vi "字符检测模板匹配.vi"(0 "Image In":T6, 1 "Image Dst":T6, 2 "ROI Descriptor (Geometric Matching 1)":T5={"Global Rectangle"=[20, 20, 890, 1177], "Contours"=[{"ID"=enum."External", "Type"=3, "Coordinates"=[20, 20, 890, 1177]}]} {"Contours"."Type" items=["No Selection", "Point", "Line", "Rectangle", "Oval", "Polygon", "Freehand Region", "Annulus", "Unused2", "Unused3", "Broken Line", "Freehand Line", "Rotated Rectangle"]}, 3 "Settings (Geometric Matching 1)":T4={"Curve Parameters"={"Extraction Mode"=0, "Edge Threshold"=75, "Edge Filter Size"=1, "Min Length"=25, "Row Search Step Size"=15, "Col Search Step Size"=15, "Max Endpoint Gap"=10, "Closed"=FALSE, "Subpixel"=FALSE}, "Match Mode"={"Rotation"=TRUE, "Scale"=FALSE, "Occlusion"=TRUE, "Reserved 1"=FALSE, "Reserved 2"=FALSE, "Reserved 3"=FALSE}, "Range Settings"=[{"Match Constraints"=0, "Min"=0.0, "Max"=360.0}, {"Match Constraints"=2, "Min"=0.0, "Max"=25.0}], "Number of Matches"=1, "Minimum Match Score"=800.0, "SubPixel Accuracy"=FALSE, "Adv. Geometric Match Options 2"=[{"Setup Data Item"=21, "Item Value"=0.0}, {"Setup Data Item"=22, "Item Value"=1.0}]} {"Curve Parameters"."Extraction Mode" items=["Normal", "Uniform Regions"]; "Curve Parameters"."Edge Filter Size" items=["Fine", "Normal", "Contour Tracing"]; "Curve Parameters"."Max Endpoint Gap" min=0; "Curve Parameters"."Col Search Step Size" min=1 max=255 step=1; "Curve Parameters"."Row Search Step Size" min=1 max=255 step=1; "Curve Parameters"."Min Length" min=0; "Curve Parameters"."Edge Threshold" min=1 max=350 step=1; "Range Settings"."Max" format="%.2f"; "Range Settings"."Min" format="%.2f"; "Range Settings"."Match Constraints" items=["Rotation Angle (degrees)", "Scale Factor (%)", "Occlusion (%)"]; "Adv. Geometric Match Options 2"."Setup Data Item" items=["Curve Extraction Mode", "Curve Edge Threshold", "Curve Edge Filter Size", "Min Curve Length", "Curve Row Search Step Size", "Curve Col Search Step Size", "Curve Max Endpoint Gap", "Extract Closed Curves", "Enable Subpixel Curve Extraction", "Enable Correlation Score", "Enable Subpixel Accuracy", "Subpixel Iterations", "Subpixel Tolerance", "Initial Match List Length", "Enable Target Template Curve Score", "Min Match Separation Distance", "Min Match Separation Angle", "Min Match Separation Scale", "Max Match Overlap", "Enable Coarse Result", "Enable Calibration Support", "Enable Contrast Reversal", "Search Strategy", "Refinement Match Factor", "Subpixel Match Factor"]}, 4 "Template File Path (Geometric Matching 1)":path=path "D:/Inspect System/Source Code/SubVIs/字符检测VI/aaaa.png", 5 "Reference System":T1 {"Axis Reference" items=["Direct", "Indirect"]; "Angle (deg)" format="%.2f"; "Origin"."Y" format="%.2f"; "Origin"."X" format="%.2f"}, 7 "error in":errorcluster) -> (20 "Image Out":T6, 21 "Matches (Geometric Matching 1)":T8[](array[typedef]) {"Correlation Score" format="%.2f"; "Target Template Curve Score" format="%.2f"; "Template Target Curve Score" format="%.2f"; "Bounding Box"."y" format="%.2f"; "Bounding Box"."x" format="%.2f"; "Position"."y" format="%.2f"; "Position"."x" format="%.2f"; "Score" format="%.2f"; "Scale" format="%.2f"; "Angle" format="%.2f"; "Occlusion %" format="%.2f"}, 22 "Calibrated Matches (Geometric Matching 1)":T8[](array[typedef]) {"Correlation Score" format="%.2f"; "Target Template Curve Score" format="%.2f"; "Template Target Curve Score" format="%.2f"; "Bounding Box"."y" format="%.2f"; "Bounding Box"."x" format="%.2f"; "Position"."y" format="%.2f"; "Position"."x" format="%.2f"; "Score" format="%.2f"; "Scale" format="%.2f"; "Angle" format="%.2f"; "Occlusion %" format="%.2f"}, 23 "Number of Matches (Geometric Matching 1)":i32, 24 "Coordinate System Out (Set Coordinate System 1)":T7 {"Measurement System"."Axis Reference" items=["Direct", "Indirect"]; "Measurement System"."Angle (deg)" format="%.2f"; "Measurement System"."Origin"."Y" format="%.2f"; "Measurement System"."Origin"."X" format="%.2f"; "Reference System"."Axis Reference" items=["Direct", "Indirect"]; "Reference System"."Angle (deg)" format="%.2f"; "Reference System"."Origin"."Y" format="%.2f"; "Reference System"."Origin"."X" format="%.2f"}, 27 "error out":errorcluster)   [LabVIEW 2017]
doc: "Creates, edits, and runs vision algorithms using NI Vision Assistant.\n\nWhen you place this Express VI on the block diagram, NI Vision Assistant launches. Create an algorithm using the Vision Assistant processing functions. After you create an algorithm, you can select the controls and indicators that you want to be able to programmatically set in LabVIEW. Double-click the Vision Assistant Express VI to edit the algorithm."
uses:
  <vilib>/vision/Image Controls.llb/IMAQ Image.ctl
  <vilib>/vision/Pattern Matching.llb/IMAQ GM Match Report.ctl
  <vilib>/vision/Pattern Matching.llb/IMAQ Curve Parameters.ctl
  <vilib>/vision/Pattern Matching.llb/IMAQ Match Range Setting.ctl
panel:
  # "Range"
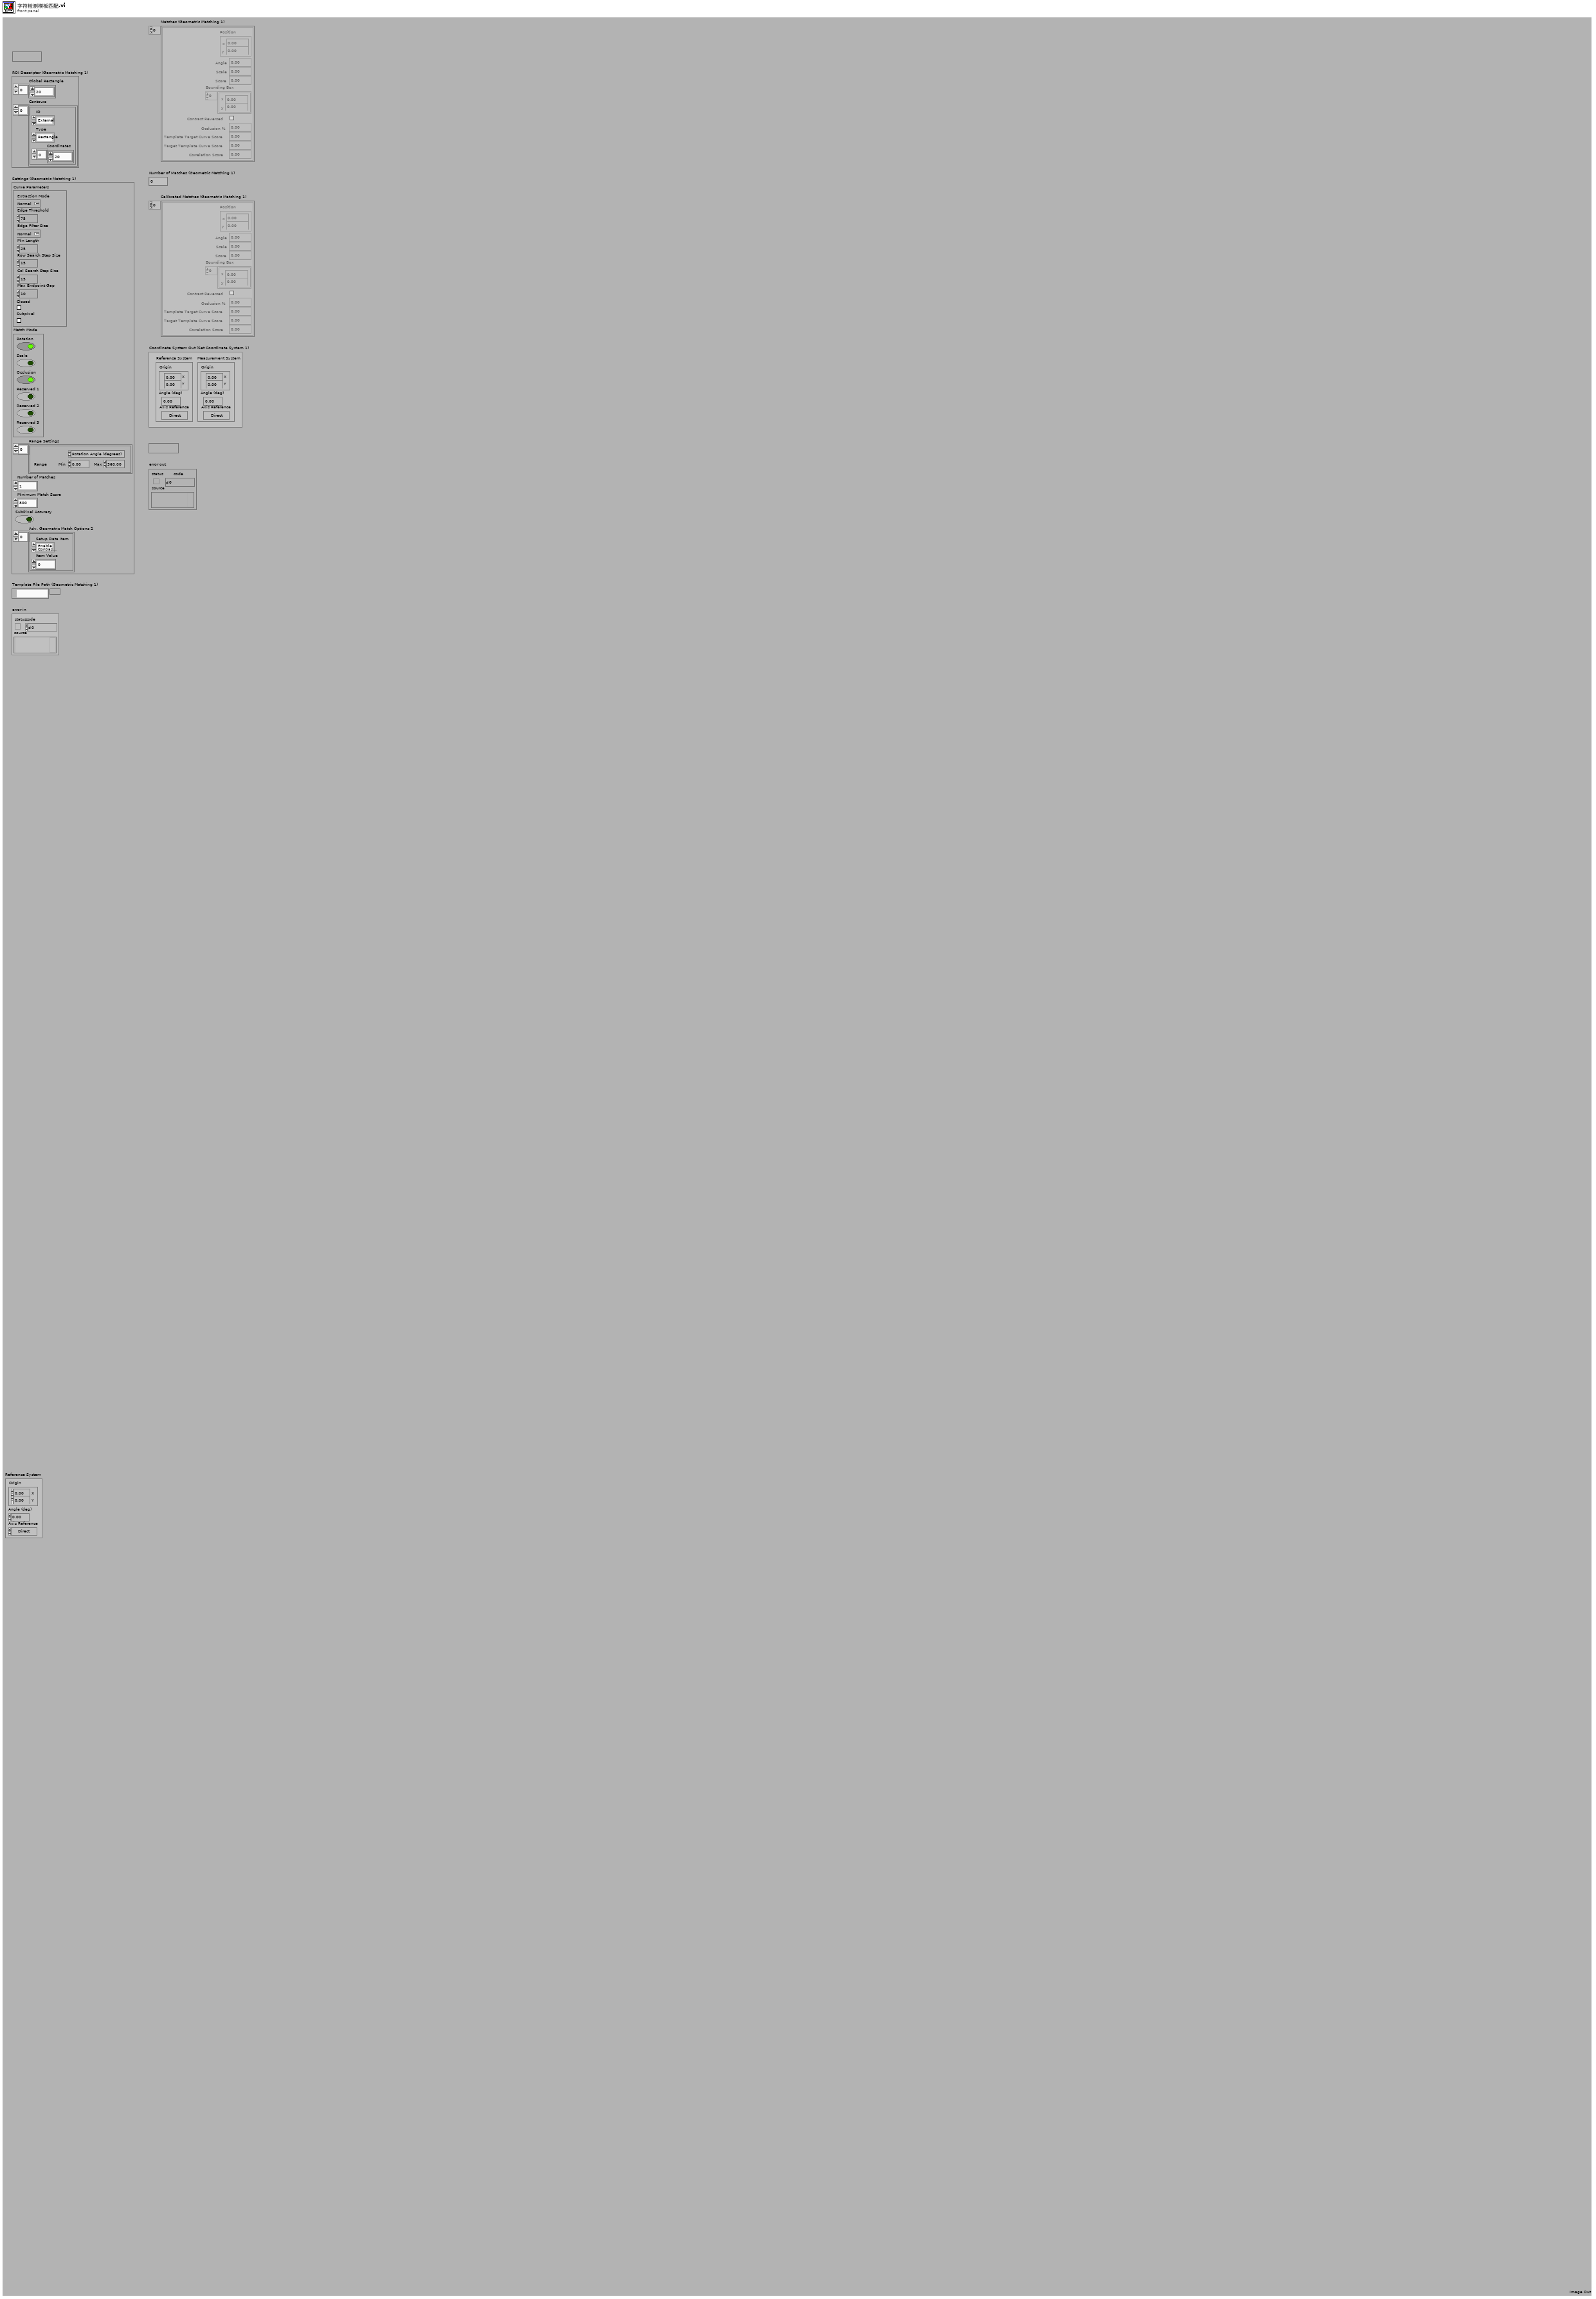
[diagram p1: front panel]
types:
  T1 = cluster{"Origin":cluster{"X":sgl, "Y":sgl}, "Angle (deg)":sgl, "Axis Reference":u32}
  T2 = typedef "IMAQ Curve Parameters.ctl" = cluster{"Extraction Mode":u32, "Edge Threshold":i32, "Edge Filter Size":u32, "Min Length":i32, "Row Search Step Size":i32, "Col Search Step Size":i32, "Max Endpoint Gap":i32, "Closed":bool, "Subpixel":bool}
  T3 = typedef "IMAQ Match Range Setting.ctl" = cluster{"Match Constraints":u32, "Min":dbl, "Max":dbl}
  T4 = cluster{"Curve Parameters":T2, "Match Mode":cluster{"Rotation":bool, "Scale":bool, "Occlusion":bool, "Reserved 1":bool, "Reserved 2":bool, "Reserved 3":bool}, "Range Settings":T3[], "Number of Matches":i32, "Minimum Match Score":sgl, "SubPixel Accuracy":bool, "Adv. Geometric Match Options 2":cluster{"Setup Data Item":u16, "Item Value":dbl}[]}
  T5 = cluster{"Global Rectangle":i32[], "Contours":cluster{"ID":enum32{"External", "Internal"}, "Type":u32, "Coordinates":i32[]}[]}
  T6 = typedef "IMAQ Image.ctl" = refnum<image>
  T7 = cluster{"Reference System":cluster{"Origin":cluster{"X":sgl, "Y":sgl}, "Angle (deg)":sgl, "Axis Reference":u32}, "Measurement System":cluster{"Origin":cluster{"X":sgl, "Y":sgl}, "Angle (deg)":sgl, "Axis Reference":u32}}
  T8 = typedef "IMAQ GM Match Report.ctl" = cluster{"Position":cluster{"x":sgl, "y":sgl}, "Angle":sgl, "Scale":sgl, "Score":sgl, "Bounding Box":cluster{"x":sgl, "y":sgl}[], "Contrast Reversed":bool, "Occlusion %":sgl, "Template Target Curve Score":sgl, "Target Template Curve Score":sgl, "Correlation Score":sgl}
  T9 = typedef "Image Type" = u32
  T10 = enum16{"Reset", "Update Coordinate System", "Get Coordinate System"}
  T11 = enum16{"Horizontal Motion", "Vertical Motion", "Horizontal and Vertical Motion", "Horizontal, Vertical and Angular Motion"}
  T12 = typedef "IMAQ Coordinate System" = cluster{"Reference System":cluster{"Origin":cluster{"X":sgl, "Y":sgl}, "Angle (deg)":sgl, "Axis Reference":u32}, "Measurement System":cluster{"Origin":cluster{"X":sgl, "Y":sgl}, "Angle (deg)":sgl, "Axis Reference":u32}}
  T13 = cluster{"Backup Image Name":string, "Coordinate System Out":T12}
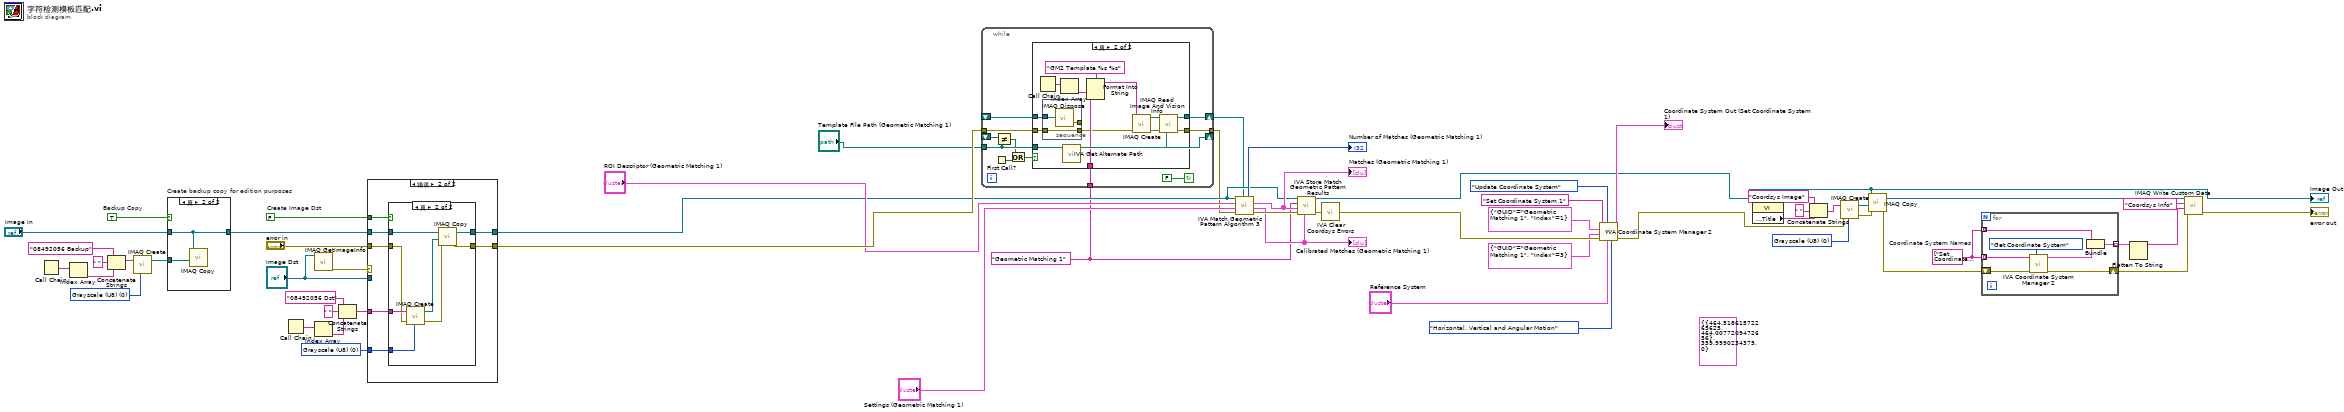
[diagram p0: block diagram]
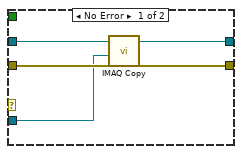
[diagram p3: hidden frame]
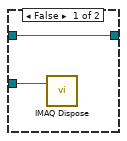
[diagram p5: hidden frame]
diagram:
  w5 = T9 0 items=["Grayscale (U8)", "Grayscale (I16)", "Grayscale (SGL)", "Complex (CSG)", "RGB (U32)", "HSL (U32)", "RGB (U64)", "Grayscale (U16)"] ("Image Type")
  w12 = string[] ["Set Coordinate System 1"]  # Coordinate System Names
  (unwired) T1 {"Origin"={"X"=464.51862, "Y"=464.00772}, "Angle (deg)"=359.99902, "Axis Reference"=0} ("Reference System")
  w29 = "Geometric Matching 1" ("Step Name")
  w38 = T9 0 items=["Grayscale (U8)", "Grayscale (I16)", "Grayscale (SGL)", "Complex (CSG)", "RGB (U32)", "HSL (U32)", "RGB (U64)", "Grayscale (U16)"] ("Image Dst Type")
  w39 = T9 0 items=["Grayscale (U8)", "Grayscale (I16)", "Grayscale (SGL)", "Complex (CSG)", "RGB (U32)", "HSL (U32)", "RGB (U64)", "Grayscale (U16)"] ("Image Type")
  w58 = TRUE  # Backup Copy
  w51 = FALSE  # Create Image Dst
  n1 = Call Chain() -> (call chain=w45:string[])
  n2 = Index Array(array=w45) -> (element=w44:string)  [unwired: 1 in]
  n3 = Concatenate Strings("08492056 Backup" ("Backup Image Name"), " ", w44) -> (w41:string)
  n4 = call "IMAQ Create"("Image Name"=w41, "Image Type"=w39) -> ("New Image"=w40:T6)  [unwired: 2 in, 2 out]
  n5 = case "Create backup copy for edition purposes" shown="真" w58 {
    tunnel: [w60 w62] -> w54
    tunnel: "Image In" -> [w60 w62]
    tunnel: w40 -> [w59 w61]
    frame False {
      n6 = call "IMAQ Dispose"("Image"=w59) -> ()  [unwired: 2 in, 4 out]
    }
    frame True {
      n7 = call "IMAQ Copy"("Image Dst"=w61, "Image Src"=w62) -> ()  [unwired: 1 in, 5 out]
    }
  }
  n8 = Call Chain() -> (call chain=w50:string[])
  n9 = call "IMAQ GetImageInfo"("Image"="Image Dst") -> ("error out"=w56:errorcluster)  [unwired: 1 in, 9 out]
  n10 = Index Array(array=w50) -> (element=w48:string)  [unwired: 1 in]
  n11 = Concatenate Strings("08492056 Dst" ("Image Dst Name"), " ", w48) -> (w46:string)
  n12 = case "条件结构" shown="错误" w56 {
    tunnel: [w67 w71] -> w31
    tunnel: [w66 w70] -> w52
    tunnel: w54 -> [w65 w72]
    tunnel: "error in" -> [w64 w68]
    tunnel: "Image Dst" -> [w63 _]
    tunnel: w46 -> [_ w74]
    tunnel: w38 -> [_ w73]
    tunnel: w51 -> [_ w69]
    frame No Error {
      n13 = call "IMAQ Copy"("error in (no error)"=w64, "Image Dst"=w63, "Image Src"=w65) -> ("error out"=w66:errorcluster, "Image Dst Out"=w67:T6)  [unwired: 3 out]
    }
    frame Error {
      n14 = case "条件结构" shown="真" w69 {
        tunnel: w74 -> [_ w84]
        tunnel: w73 -> [_ w83]
        tunnel: w72 -> [w76 w81]
        tunnel: [w76 w80] -> w71
        tunnel: [w75 w79] -> w70
        tunnel: w68 -> [w75 w77]
        frame False {
        }
        frame True {
          n15 = call "IMAQ Create"("Image Name"=w84, "Image Type"=w83, "error in (no error)"=w77) -> ("New Image"=w82:T6, "error out"=w78:errorcluster)  [unwired: 1 in, 1 out]
          n16 = call "IMAQ Copy"("error in (no error)"=w78, "Image Dst"=w82, "Image Src"=w81) -> ("error out"=w79:errorcluster, "Image Dst Out"=w80:T6)  [unwired: 3 out]
        }
      }
    }
  }
  n17 = while {
    shift-right: [w95] -> w27
    shift-left: _ -> [w94]
    tunnel: [w92] -> w28
    tunnel: w52 -> [w91]
    tunnel: "Template File Path (Geometric Matching 1)" -> [w88]
    tunnel: w29 -> [w90]
    shift-right: [w88] -> _
    shift-left: _ -> [w89]
    stop <- FALSE continue-if-true
    n18 = First Call?() -> (First Call?: T/F=w87:bool)
    n19 = Not Equal?(x=w89, y=w88) -> (x != y?=w86:bool)
    n20 = Or(x=w86, y=w87) -> (x .or. y?=w85:bool)
    n21 = case "条件结构" shown="真" w85 {
      tunnel: [w97 w109] -> w95
      tunnel: w94 -> [w97 w101]
      tunnel: [w96 w106] -> w92
      tunnel: w91 -> [w96 w102]
      tunnel: w90 -> [_ w103]
      tunnel: w88 -> [_ w100]
      frame False {
      }
      frame True {
        n22 = Call Chain() -> (call chain=w105:string[])
        n23 = stacked-sequence "层叠式顺序结构" {
          tunnel: w102 -> [w114]
          tunnel: w101 -> [w113]
          tunnel: [w114] -> w98
          tunnel: [w112] -> _
          frame #0 {
            n24 = call "IMAQ Dispose"("Image"=w113) -> ("error out"=w112:errorcluster)  [unwired: 2 in, 3 out]
          }
        }
        n25 = Index Array(array=w105) -> (element=w104:string)  [unwired: 1 in]
        n26 = call <vilib>:"IVA Get Alternate Path.vi"("Path In"=w100) -> ("Path Out"=w99:path)  [unwired: 10 out]
        n27 = Format Into String(format string="GM2 Template %s %s" ("Image Name"), w104, w103) -> (resulting string=w111:string)  [unwired: 2 in, 1 out]
        n28 = call "IMAQ Create"("Image Name"=w111, "error in (no error)"=w98) -> ("New Image"=w108:T6, "error out"=w107:errorcluster)  [unwired: 2 in, 1 out]
        n29 = call "IMAQ Read Image And Vision Info"("File Path"=w99, "error in (no error)"=w107, "Image"=w108) -> ("error out"=w106:errorcluster, "Image Out"=w109:T6)  [unwired: 1 in, 6 out]
      }
    }
  }
  n30 = call <vilib>:"IVA Match Geometric Pattern Algorithm 3.vi"("Template"=w27, "error in (no error)"=w28, "Settings"="Settings (Geometric Matching 1)", "ROI Descriptor"="ROI Descriptor (Geometric Matching 1)", "Image"=w31) -> ("error out"=w35:errorcluster, "Calibrated Matches"=w33:T8[], "Matches"=w34:T8[], "Number of Matches"=→"Number of Matches (Geometric Matching 1)":i32)  [unwired: 3 out]
  "Matches (Geometric Matching 1)" <- w34
  "Calibrated Matches (Geometric Matching 1)" <- w33
  n31 = call <vilib>:"IVA Store Match Geometric Pattern Results.vi"("Calibrated Matches"=w33, "error in (no error)"=w35, "Matches"=w34, "Step Name"=w29, "Image in"=w31) -> ("error out"=w26:errorcluster, "Image dup"=w2:T6)  [unwired: 5 out]
  "Image Out" <- w2
  n32 = call <vilib>:"IVA Clear Coordsys Errors.vi"("error in (no error)"=w26) -> ("error out"=w25:errorcluster)  [unwired: 10 in]
  n33 = call <vilib>:"IVA Coordinate System Manager 2.vi"("Mode"=T11."Horizontal, Vertical and Angular Motion", "Reference System"="Reference System", "Function"=T10."Update Coordinate System", "error in (no error)"=w25, "Angle ID"=cluster{"GUID":string, "Index":i32} {"GUID"="Geometric Matching 1", "Index"=3}, "Origin ID"=cluster{"GUID":string, "Index":i32} {"GUID"="Geometric Matching 1", "Index"=1}, "Coordinate System Name"="Set Coordinate System 1") -> ("error out"=w19:errorcluster, "Coordinate System Out"=→"Coordinate System Out (Set Coordinate System 1)":T12)  [unwired: 3 out]
  n34 = property class="VI"() -> ("Front Panel Window:Title"=w6:string)  [unwired: 2 in, 2 out]
  n35 = Concatenate Strings("Coordsys Image" ("Processed Image Name"), " ", w6) -> (w15:string)
  n36 = call "IMAQ Create"("Image Name"=w15, "Image Type"=w5, "error in (no error)"=w19) -> ("New Image"=w13:T6, "error out"=w14:errorcluster)  [unwired: 1 in, 1 out]
  n37 = call "IMAQ Copy"("error in (no error)"=w14, "Image Dst"=w13, "Image Src"=w2) -> ("error out"=w4:errorcluster, "Image Dst Out"=w11:T6)  [unwired: 3 out]
  n38 = for "For循环" {
    tunnel: w12 -> [w120] mode=indexing
    tunnel: w12 -> [w118] mode=indexing
    tunnel: [w117] -> w10 mode=indexing
    shift-right: [w115] -> w3
    shift-left: w4 -> [w116]
    n39 = call <vilib>:"IVA Coordinate System Manager 2.vi"("Function"=T10."Get Coordinate System", "error in (no error)"=w116, "Coordinate System Name"=w120) -> ("error out"=w115:errorcluster, "Coordinate System Out"=w119:T12)  [unwired: 4 in, 3 out]
    n40 = Bundle("Backup Image Name"=w118, "Coordinate System Out"=w119) -> (w117:T13)  [unwired: 1 out]
  }
  n41 = Flatten To String(anything=w10) -> (data string=w9:string)  [unwired: 1 in, 4 out]
  n42 = call "IMAQ Write Custom Data"("error in (no error)"=w3, "Custom Data In"=w9, "Key"="Coordsys Info", "Image"=w11) -> ("error out"=→"error out":errorcluster)  [unwired: 7 out]
